vi "HP81110A Query Arm Source.vi"(8 "error in (no error)":errorcluster, 11 "VISA session":refnum<visa-resource-name>) -> (0 "error out":errorcluster, 2 "Arming (Trigger) Source (0:Internal PLL)":T1(ring)=enum."External", 3 "dup VISA session":refnum<visa-resource-name>)   [LabVIEW 2017]
doc: "This VI queries the arming (triggering) source. Results can be:\n0 = Immediate (internal oscillator)\n1 = Internal PLL\n2 = External \n3 = Manual"
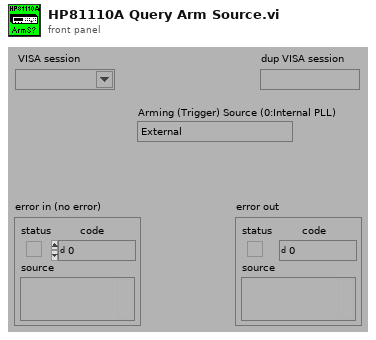
[diagram p1: front panel]
types:
  T1 = enum16{"Immediate (Continuous Mode)", "Internal PLL", "External", "Manual"}
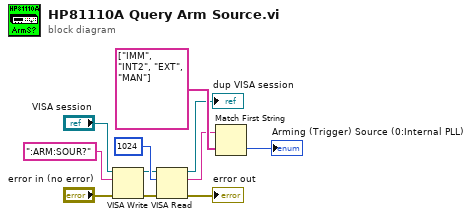
[diagram p0: block diagram]
diagram:
  n1 = VISA Write(VISA resource name="VISA session", write buffer=":ARM:SOUR?", error in (no error)="error in (no error)") -> (VISA resource name out=w5:refnum<visa-resource-name>, error out=w6:errorcluster)  [unwired: 1 out]
  n2 = VISA Read(VISA resource name=w5, byte count=u32 1024 ("byte count (0)"), error in (no error)=w6) -> (VISA resource name out=→"dup VISA session":refnum<visa-resource-name>, read buffer=w7:string, error out=→"error out":errorcluster)  [unwired: 1 out]
  n3 = Match First String(2:string[] ["IMM", "INT2", "EXT", "MAN"] ("string array"), 3:w7) -> (0:→"Arming (Trigger) Source (0:Internal PLL)":i32)  [unwired: 1 out]
